vi "Moving Average.vi"   [LabVIEW 2016, in "xy_utilities.lvlib"]
doc: "Apply a moving average <b>XY-data</b>'s Y-Array according to <b>window</b>.\n\nWire data to the data input to determine the polymorphic instance to use or manually select the instance."
uses:
  xy_utilities.lvlib
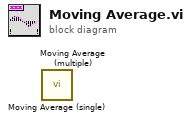
[diagram p0: block diagram]
diagram:
  n1 = call "Moving Average (single).vi"() -> ()  [unwired: 10 in, 2 out]
  n2 = call "Moving Average (multiple).vi"() -> ()  [unwired: 10 in, 2 out]
